vi "pathVI.vi"(7 "gap":i32=5, 11 "ROI":T1={"Global Rectangle"=[28, 22, 307, 232], "Contours"=[{"Contour Type"=0, "ROI Type"=11, "Points"=[55, 203, 57, 204, 60, 205, 63, 207, 67, 210, 73, 212, 80, 215, 86, 218, 93, 221, 102, 224, 109, 227, 117, 229, 124, 230, 132, 231, 139, 231, 144, 231, 151, 230, 157, 229, 164, 228, 172, 227, 180, 226, 188, 225, 196, 224, 203, 223, 209, 222, 213, 221, 216, 221, 217, 221, 217, 220, 217, 219, 219, 218, 221, 216, 223, 214, 225, 211, 227, 208, 229, 205, 231, 200, 231, 197, 232, 193, 233, 190, 234, 187, 235, 184, 235, 182, 235, 180, 234, 179, 233, 178, 232, 177, 232, 176, 231, 176, 230, 175, 228, 175, 226, 175, 224, 175, 219, 175, 214, 175, 206, 176, 196, 176, 187, 177, 176, 178, 167, 179, 160, 180, 156, 180, 153, 180, 151, 180, 150, 180, 148, 180, 144, 180, 141, 180, 138, 179, 133, 178, 127, 177, 121, 175, 116, 172, 107, 169, 99, 166, 92, 164, 83, 161, 77, 158, 74, 156, 72, 155, 71, 155, 70, 154, 69, 153, 69, 152, 68, 152, 68, 151, 67, 150, 67, 148, 67, 146, 67, 144, 67, 141, 70, 139, 72, 137, 74, 134, 78, 132, 82, 129, 88, 126, 94, 123, 102, 122, 112, 122, 121, 122, 133, 122, 146, 122, 158, 123, 170, 124, 182, 125, 197, 128, 214, 129, 232, 130, 246, 131, 257, 131, 264, 131, 269, 131, 273, 130, 277, 130, 279, 128, 280, 127, 282, 125, 282, 123, 283, 121, 284, 119, 285, 116, 285, 112, 286, 109, 287, 106, 288, 103, 288, 100, 289, 97, 290, 94, 290, 91, 290, 88, 289, 85, 288, 82, 286, 79, 285, 77, 283, 75, 281, 73, 279, 71, 275, 68, 270, 66, 263, 63, 255, 62, 246, 61, 234, 59, 224, 59, 211, 61, 199, 61, 187, 61, 174, 61, 162, 59, 150, 58, 139, 58, 128, 57, 119, 57, 111, 58, 102, 59, 93, 59, 85, 59, 77, 59, 69, 59, 61, 59, 53, 58, 46, 57, 41, 56, 35, 56, 32, 55, 31, 54, 29, 53, 28, 53, 28, 52, 28, 51, 28, 50, 29, 49, 29, 48, 30, 47, 31, 46, 32, 45, 32, 44, 33, 44, 33, 43, 34, 43, 34, 42, 35, 42, 35, 41, 36, 40, 38, 38, 39, 37, 40, 37, 42, 36, 44, 35, 46, 34, 48, 34, 51, 33, 54, 32, 57, 32, 60, 31, 63, 31, 66, 31, 69, 31, 72, 31, 77, 31, 83, 32, 92, 31, 101, 30, 112, 29, 121, 29, 129, 28, 137, 28, 143, 28, 147, 28, 150, 27, 152, 27, 154, 27, 156, 27, 159, 27, 161, 27, 164, 27, 167, 27, 169, 27, 172, 27, 175, 27, 180, 27, 184, 27, 189, 27, 195, 27, 201, 26, 206, 26, 210, 25, 214, 25, 219, 24, 222, 23, 224, 23, 225, 22, 227, 22, 228, 22, 229, 22, 230, 22, 231, 22, 233, 22, 235, 22, 237, 23, 240, 24, 242, 25, 245, 25, 246, 25, 247, 26, 248, 27, 249, 27, 250, 28, 252, 28, 254, 29, 256, 30, 258, 30, 259, 31, 261, 31, 262, 32, 264, 32, 265, 32, 267, 33, 269, 33, 270, 33, 272, 34, 273, 35, 274, 35, 275, 35, 277, 36, 278, 36, 279, 37, 280, 37, 281, 37, 282, 37, 283, 37, 284, 37, 285, 37, 286, 37, 287, 37, 287, 36, 288, 36, 289, 36, 290, 36, 291, 35, 292, 34, 293, 33, 294, 33, 294, 32, 295, 32, 295, 31, 296, 31, 296, 30, 297, 30, 298, 30, 299, 30, 300, 30, 301, 30, 302, 29, 303, 29, 304, 29, 304, 28, 305, 28, 306, 28, 306, 28]}]}) -> (3 "Array":cluster{i32, i32}[](array[cluster]))   [LabVIEW 2015]
panel:
  out "x-1":i32
  out "size(s)":i32
  out "Points":i32[](array[numeric])
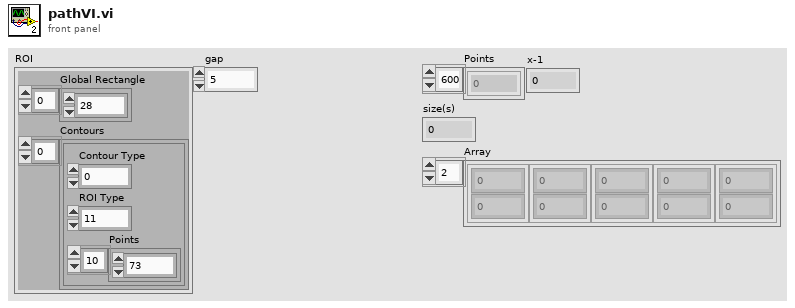
[diagram p1: front panel]
types:
  T1 = cluster{"Global Rectangle":i32[], "Contours":cluster{"Contour Type":u32, "ROI Type":u32, "Points":i32[]}[]}
  T2 = cluster{"Contour Type":u32, "ROI Type":u32, "Points":i32[]}[]
  T3 = cluster{"Contour Type":u32, "ROI Type":u32, "Points":i32[]}
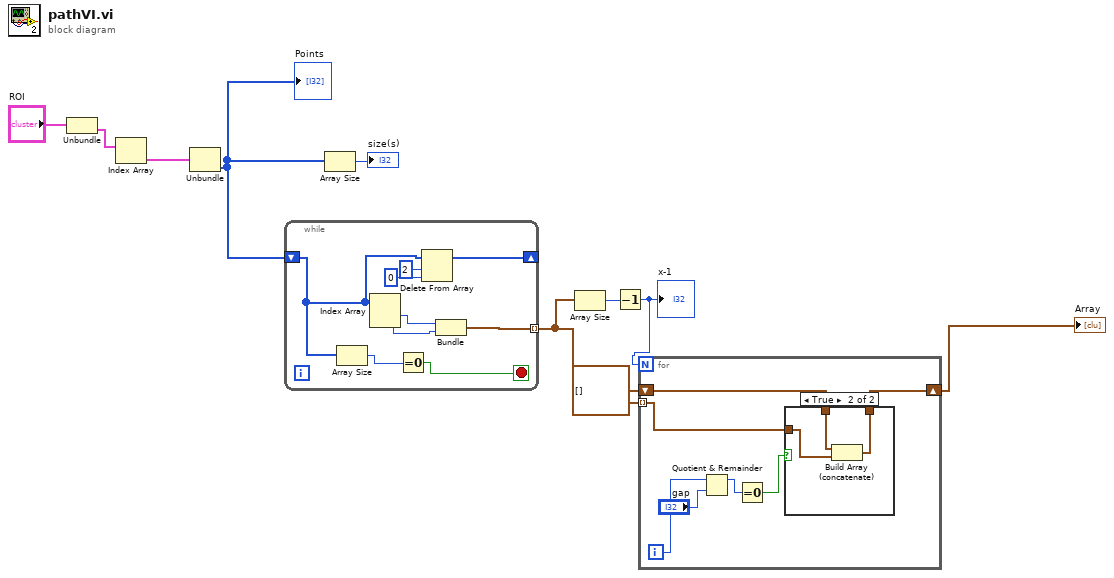
[diagram p0: block diagram]
diagram:
  n1 = Unbundle("ROI") -> ("Contours"=w9:T2)  [unwired: 1 out]
  n2 = Index Array(array=w9) -> (element=w8:T3)  [unwired: 1 in]
  n3 = Unbundle(w8) -> ("Points"=w6:i32[])  [unwired: 2 out]
  "Points" <- w6
  n4 = while {
    shift-right: [w16] -> _
    shift-left: w6 -> [w14]
    tunnel: [w15] -> w3 mode=indexing
    stop <- w12 stop-if-true
    n5 = Array Size(array=w14) -> (size(s)=w13:i32)
    n6 = Index Array(array=w14) -> (element #1=w19:i32, element #2=w18:i32)  [unwired: 2 in]
    n7 = Equal To 0?(x=w13) -> (x = 0?=w12:bool)
    n8 = Delete From Array(array=w14, length=2, index=0) -> (array with subset deleted=w16:i32[])  [unwired: 1 out]
    n9 = Bundle(w19, w18) -> (w15:cluster{i32, i32})  [unwired: 1 in]
  }
  n10 = Array Size(array=w6) -> (size(s)=→"size(s)":i32)
  n11 = Array Size(array=w3) -> (size(s)=w2:i32)
  n12 = Decrement(x=w2) -> (x-1=w1:i32)
  "x-1" <- w1
  n13 = for {
    N: w1 -> [_]
    tunnel: w3 -> [w22] mode=indexing
    shift-right: [w21] -> w5
    shift-left: cluster{i32, i32}[] [] -> [w20]
    i -> [w26]
    n14 = Quotient & Remainder(x=w26, y="gap") -> (x-y*floor(x/y)=w23:i32)  [unwired: 1 out]
    n15 = Equal To 0?(x=w23) -> (x = 0?=w25:bool)
    n16 = case shown="True" w25 {
      tunnel: w22 -> [_ w30]
      tunnel: [w27 w29] -> w21
      tunnel: w20 -> [w27 w28]
      frame False {
      }
      frame True {
        n17 = Build Array (concatenate)(w28, w30) -> (w29:cluster{i32, i32}[])
      }
    }
  }
  "Array" <- w5
